vi "ConfigChannels.vi"(8 "error in (no error)":errorcluster, 11 "DigitizerBase in":refnum<class "DigitizerBase.lvclass">) -> (0 "error out":errorcluster, 3 "DigitizerBase out":refnum<class "DigitizerBase.lvclass">)   [LabVIEW 2014, in "DigitizerPlugins.lvlib" / "DigitizerBase.lvclass"]
uses:
  DigitizerBase.lvclass
  DigitizerBase.lvclass/DigitizerBase.ctl
  Accessors/Write InstRef.vi
  Accessors/Read InstRef.vi
  Accessors/Read Channels.vi
  <vilib>/Utility/error.llb/Error Cluster From Error Code.vi
  <vilib>/ErrorRing/Error Ring.xnode
panel:
  in  "Name":string
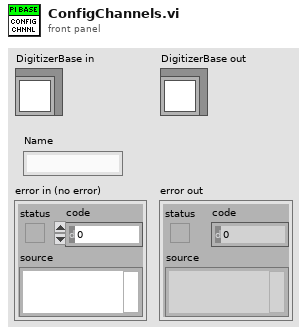
[diagram p1: front panel]
types:
  T1 = typedef "DigitizerPlugins.lvlib/DigitizerBase.lvclass/Channel.ctl" = cluster{"Name":string, "Enabled":bool, "InputImpedance":dbl, "Coupling":enum16{"AC", "DC", "Gnd"}, "Offset":dbl, "Range":dbl}
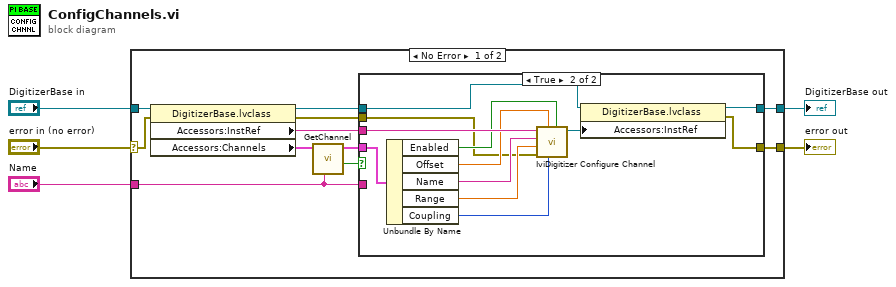
[diagram p0: block diagram]
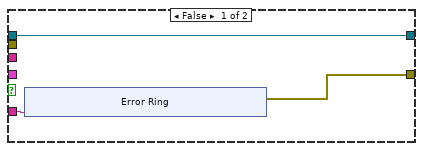
[diagram p2: hidden frame]
diagram:
  n1 = case shown="No Error" "error in (no error)" {
    selector: "error in (no error)" -> [w15 w40]
    tunnel: [w9 w40] -> w4
    tunnel: [w7 w39] -> w2
    tunnel: "DigitizerBase in" -> [w16 w39]
    tunnel: "Name" -> [w10 _]
    frame No Error {
      n2 = property class="DigitizerBase.lvclass"(reference=w16, error in=w15) -> (reference out=w8:refnum<class "DigitizerBase.lvclass">, error out=w6:errorcluster, "Accessors:InstRef"=w12:string, "Accessors:Channels"=w14:T1[])
      n3 = call "GetChannel.vi"("Name"=w10, "Channels"=w14) -> ("Channel"=w11:T1, "Found?"=w13:bool)  [unwired: 8 in]
      n4 = case shown="True" w13 {
        tunnel: w12 -> [_ w38]
        tunnel: w11 -> [_ w37]
        tunnel: w10 -> [w19 _]
        tunnel: [w18 w27] -> w9
        tunnel: w8 -> [w17 w30]
        tunnel: [w17 w28] -> w7
        tunnel: w6 -> [_ w31]
        frame False {
          n5 = xnode "Error Ring"("parameter 0"=w19) -> ("error out"=w18:errorcluster)
        }
        frame True {
          n6 = Unbundle By Name(w37) -> ("Enabled"=w36:bool, "Offset"=w35:dbl, "Name"=w34:string, "Range"=w33:dbl, "Coupling"=w32:enum16{"AC", "DC", "Gnd"})
          n7 = call <vilib>:"IviDigitizer Configure Channel.vi"("Channel Enabled (Off)"=w36, "Vertical Coupling (AC Coupling)"=w32, "Vertical Offset (0.0)"=w35, "error in (no error)"=w31, "Vertical Range (1.0)"=w33, "Channel Name (\"\")"=w34, "instrument handle"=w38) -> ("instrument handle out"=w29:refnum<k15>)  [unwired: 3 in, 1 out]
          n8 = property class="DigitizerBase.lvclass"(reference=w30, "Accessors:InstRef"=w29) -> (reference out=w28:refnum<class "DigitizerBase.lvclass">, error out=w27:errorcluster)  [unwired: 1 in]
        }
      }
    }
    frame Error {
    }
  }
  "error out" <- w4
  "DigitizerBase out" <- w2
